vi "rszvl_core_global.vi"() -> ()   [LabVIEW 2014] (continued)
  in  "Range Tables":T3(array[cluster])=[{"Name"="rszvl_rngUnits", "Type"=2, "Min?"=FALSE, "Max?"=FALSE, "Entries"=[{"Name"="RSZVL_VAL_UNIT_DBM", "Discrete or Min"=0.0, "Max"=0.0, "Coerced"=0.0, "Command"="DBM"}, {"Name"="RSZVL_VAL_UNIT_DBPW", "Discrete or Min"=1.0, "Max"=0.0, "Coerced"=0.0, "Command"="DBPW"}, {"Name"="RSZVL_VAL_UNIT_WATT", "Discrete or Min"=2.0, "Max"=0.0, "Coerced"=0.0, "Command"="WATT"}, {"Name"="RSZVL_VAL_UNIT_DBUV", "Discrete or Min"=3.0, "Max"=0.0, "Coerced"=0.0, "Command"="DBUV"}, {"Name"="RSZVL_VAL_UNIT_DBMV", "Discrete or Min"=4.0, "Max"=0.0, "Coerced"=0.0, "Command"="DBMV"}, {"Name"="RSZVL_VAL_UNIT_VOLT", "Discrete or Min"=5.0, "Max"=0.0, "Coerced"=0.0, "Command"="VOLT"}, {"Name"="RSZVL_VAL_UNIT_DBUA", "Discrete or Min"=6.0, "Max"=0.0, "Coerced"=0.0, "Command"="DBUA"}, {"Name"="RSZVL_VAL_UNIT_AMP", "Discrete or Min"=7.0, "Max"=0.0, "Coerced"=0.0, "Command"="AMP"}, {"Name"="RSZVL_VAL_UNIT_DB", "Discrete or Min"=8.0, "Max"=0.0, "Coerced"=0.0, "Command"="DB"}, {"Name"="RSZVL_VAL_UNIT_DEG", "Discrete or Min"=9.0, "Max"=0.0, "Coerced"=0.0, "Command"="DEG"}, {"Name"="RSZVL_VAL_UNIT_RAD", "Discrete or Min"=10.0, "Max"=0.0, "Coerced"=0.0, "Command"="RAD"}, {"Name"="RSZVL_VAL_UNIT_S", "Discrete or Min"=11.0, "Max"=0.0, "Coerced"=0.0, "Command"="S"}, {"Name"="RSZVL_VAL_UNIT_HZ", "Discrete or Min"=12.0, "Max"=0.0, "Coerced"=0.0, "Command"="HZ"}, {"Name"="RSZVL_VAL_UNIT_PCT", "Discrete or Min"=13.0, "Max"=0.0, "Coerced"=0.0, "Command"="PCT"}, {"Name"="RSZVL_VAL_UNIT_UNITLESS", "Discrete or Min"=14.0, "Max"=0.0, "Coerced"=0.0, "Command"="UNIT"}, {"Name"="RSZVL_VAL_UNIT_DBPT", "Discrete or Min"=15.0, "Max"=0.0, "Coerced"=0.0, "Command"="DBPT"}]}, {"Name"="rszvl_rngTraceMode", "Type"=2, "Min?"=FALSE, "Max?"=FALSE, "Entries"=[{"Name"="RSZVL_TRAC_MOD_WRITE", "Discrete or Min"=0.0, "Max"=0.0, "Coerced"=0.0, "Command"="WRIT"}, {"Name"="RSZVL_TRAC_MOD_VIEW", "Discrete or Min"=1.0, "Max"=0.0, "Coerced"=0.0, "Command"="VIEW"}, {"Name"="RSZVL_TRAC_MOD_AVER", "Discrete or Min"=2.0, "Max"=0.0, "Coerced"=0.0, "Command"="AVER"}, {"Name"="RSZVL_TRAC_MOD_MAXH", "Discrete or Min"=3.0, "Max"=0.0, "Coerced"=0.0, "Command"="MAXH"}, {"Name"="RSZVL_TRAC_MOD_MINH", "Discrete or Min"=4.0, "Max"=0.0, "Coerced"=0.0, "Command"="MINH"}, {"Name"="RSZVL_TRAC_MOD_BLANK", "Discrete or Min"=5.0, "Max"=0.0, "Coerced"=0.0, "Command"="BLAN"}]}, {"Name"="rszvl_rngAmplitudeUnitsRangeTable", "Type"=2, "Min?"=FALSE, "Max?"=FALSE, "Entries"=[{"Name"="RSZVL_VAL_AMPLITUDE_UNITS_DBM", "Discrete or Min"=0.0, "Max"=0.0, "Coerced"=0.0, "Command"="DBM"}, {"Name"="RSZVL_VAL_AMPLITUDE_UNITS_DBMV", "Discrete or Min"=1.0, "Max"=0.0, "Coerced"=0.0, "Command"="DBMV"}, {"Name"="RSZVL_VAL_AMPLITUDE_UNITS_DBUV", "Discrete or Min"=2.0, "Max"=0.0, "Coerced"=0.0, "Command"="DBUV"}, {"Name"="RSZVL_VAL_AMPLITUDE_UNITS_VOLT", "Discrete or Min"=3.0, "Max"=0.0, "Coerced"=0.0, "Command"="V"}, {"Name"="RSZVL_VAL_AMPLITUDE_UNITS_WATT", "Discrete or Min"=4.0, "Max"=0.0, "Coerced"=0.0, "Command"="W"}, {"Name"="RSZVL_VAL_AMPLITUDE_UNITS_DBPW", "Discrete or Min"=5.0, "Max"=0.0, "Coerced"=0.0, "Command"="DBPW"}, {"Name"="RSZVL_VAL_AMPLITUDE_UNITS_DBUA", "Discrete or Min"=6.0, "Max"=0.0, "Coerced"=0.0, "Command"="DBUA"}, {"Name"="RSZVL_VAL_AMPLITUDE_UNITS_AMP", "Discrete or Min"=7.0, "Max"=0.0, "Coerced"=0.0, "Command"="A"}]}, {"Name"="rszvl_rngAbsRel", "Type"=2, "Min?"=FALSE, "Max?"=FALSE, "Entries"=[{"Name"="RSZVL_VAL_ABS", "Discrete or Min"=0.0, "Max"=0.0, "Coerced"=0.0, "Command"="ABS"}, {"Name"="RSZVL_VAL_REL", "Discrete or Min"=1.0, "Max"=0.0, "Coerced"=0.0, "Command"="REL"}]}, {"Name"="rszvl_rngESPMode", "Type"=2, "Min?"=FALSE, "Max?"=FALSE, "Entries"=[{"Name"="RSZVL_VAL_ESP_MODE_AUTO", "Discrete or Min"=0.0, "Max"=0.0, "Coerced"=0.0, "Command"="AUTO"}, {"Name"="RSZVL_VAL_ESP_MODE_MAN", "Discrete or Min"=1.0, "Max"=0.0, "Coerced"=0.0, "Command"="MAN"}, {"Name"="RSZVL_VAL_ESP_MODE_USER", "Discrete or Min"=2.0, "Max"=0.0, "Coerced"=0.0, "Command"="USER"}]}, {"Name"="rszvl_rngDetectorTypeRangeTable", "Type"=2, "Min?"=FALSE, "Max?"=FALSE, "Entries"=[{"Name"="RSZVL_VAL_DETECTOR_TYPE_AUTO_PEAK", "Discrete or Min"=0.0, "Max"=0.0, "Coerced"=0.0, "Command"="APE"}, {"Name"="RSZVL_VAL_DETECTOR_TYPE_AVERAGE", "Discrete or Min"=1.0, "Max"=0.0, "Coerced"=0.0, "Command"="AVER"}, {"Name"="RSZVL_VAL_DETECTOR_TYPE_MAX_PEAK", "Discrete or Min"=2.0, "Max"=0.0, "Coerced"=0.0, "Command"="POS"}, {"Name"="RSZVL_VAL_DETECTOR_TYPE_MIN_PEAK", "Discrete or Min"=3.0, "Max"=0.0, "Coerced"=0.0, "Command"="NEG"}, {"Name"="RSZVL_VAL_DETECTOR_TYPE_SAMPLE", "Discrete or Min"=4.0, "Max"=0.0, "Coerced"=0.0, "Command"="SAMP"}, {"Name"="RSZVL_VAL_DETECTOR_TYPE_RMS", "Discrete or Min"=5.0, "Max"=0.0, "Coerced"=0.0, "Command"="RMS"}, {"Name"="RSZVL_VAL_DETECTOR_TYPE_QPK", "Discrete or Min"=6.0, "Max"=0.0, "Coerced"=0.0, "Command"="QPE"}]}, {"Name"="rszvl_rngDISPConfPreDefColour", "Type"=2, "Min?"=FALSE, "Max?"=FALSE, "Entries"=[{"Name"="RSZVL_VAL_DISP_COL_BLAC", "Discrete or Min"=0.0, "Max"=0.0, "Coerced"=0.0, "Command"="BLAC"}, {"Name"="RSZVL_VAL_DISP_COL_BLUE", "Discrete or Min"=1.0, "Max"=0.0, "Coerced"=0.0, "Command"="BLUE"}, {"Name"="RSZVL_VAL_DISP_COL_BROW", "Discrete or Min"=2.0, "Max"=0.0, "Coerced"=0.0, "Command"="BROW"}, {"Name"="RSZVL_VAL_DISP_COL_GRE", "Discrete or Min"=3.0, "Max"=0.0, "Coerced"=0.0, "Command"="GRE"}, {"Name"="RSZVL_VAL_DISP_COL_CYAN", "Discrete or Min"=4.0, "Max"=0.0, "Coerced"=0.0, "Command"="CYAN"}, {"Name"="RSZVL_VAL_DISP_COL_RED", "Discrete or Min"=5.0, "Max"=0.0, "Coerced"=0.0, "Command"="RED"}, {"Name"="RSZVL_VAL_DISP_COL_MAG", "Discrete or Min"=6.0, "Max"=0.0, "Coerced"=0.0, "Command"="MAG"}, {"Name"="RSZVL_VAL_DISP_COL_YELL", "Discrete or Min"=7.0, "Max"=0.0, "Coerced"=0.0, "Command"="YELL"}, {"Name"="RSZVL_VAL_DISP_COL_WHIT", "Discrete or Min"=8.0, "Max"=0.0, "Coerced"=0.0, "Command"="WHIT"}, {"Name"="RSZVL_VAL_DISP_COL_DGRA", "Discrete or Min"=9.0, "Max"=0.0, "Coerced"=0.0, "Command"="DGR"}, {"Name"="RSZVL_VAL_DISP_COL_LGRA", "Discrete or Min"=10.0, "Max"=0.0, "Coerced"=0.0, "Command"="LGR"}, {"Name"="RSZVL_VAL_DISP_COL_LBLU", "Discrete or Min"=11.0, "Max"=0.0, "Coerced"=0.0, "Command"="LBL"}, {"Name"="RSZVL_VAL_DISP_COL_LGRE", "Discrete or Min"=12.0, "Max"=0.0, "Coerced"=0.0, "Command"="LGR"}, {"Name"="RSZVL_VAL_DISP_COL_LCY", "Discrete or Min"=13.0, "Max"=0.0, "Coerced"=0.0, "Command"="LCY"}, {"Name"="RSZVL_VAL_DISP_COL_LRED", "Discrete or Min"=14.0, "Max"=0.0, "Coerced"=0.0, "Command"="LRED"}, {"Name"="RSZVL_VAL_DISP_COL_LMAG", "Discrete or Min"=15.0, "Max"=0.0, "Coerced"=0.0, "Command"="LMAG"}]}, {"Name"="rszvl_rngHcopyDeviceLang", "Type"=2, "Min?"=FALSE, "Max?"=FALSE, "Entries"=[{"Name"="RSZVL_VAL_HCOPY_DEVICE_LANG_GDI", "Discrete or Min"=0.0, "Max"=0.0, "Coerced"=0.0, "Command"="GDI"}, {"Name"="RSZVL_VAL_HCOPY_DEVICE_LANG_WMF", "Discrete or Min"=1.0, "Max"=0.0, "Coerced"=0.0, "Command"="WMF"}, {"Name"="RSZVL_VAL_HCOPY_DEVICE_LANG_EWMF", "Discrete or Min"=2.0, "Max"=0.0, "Coerced"=0.0, "Command"="EWMF"}, {"Name"="RSZVL_VAL_HCOPY_DEVICE_LANG_BMP", "Discrete or Min"=3.0, "Max"=0.0, "Coerced"=0.0, "Command"="BMP"}, {"Name"="RSZVL_VAL_HCOPY_DEVICE_LANG_JPG", "Discrete or Min"=4.0, "Max"=0.0, "Coerced"=0.0, "Command"="JPG"}, {"Name"="RSZVL_VAL_HCOPY_DEVICE_LANG_PNG", "Discrete or Min"=5.0, "Max"=0.0, "Coerced"=0.0, "Command"="PNG"}]}, {"Name"="rszvl_rngHcopyDeviceOrient", "Type"=2, "Min?"=FALSE, "Max?"=FALSE, "Entries"=[{"Name"="RSZVL_VAL_HCOPY_DEVICE_ORIENT_LAND", "Discrete or Min"=0.0, "Max"=0.0, "Coerced"=0.0, "Command"="LAND"}, {"Name"="RSZVL_VAL_HCOPY_DEVICE_ORIENT_PORT", "Discrete or Min"=1.0, "Max"=0.0, "Coerced"=0.0, "Command"="PORT"}]}, {"Name"="rszvl_rngDomain", "Type"=2, "Min?"=FALSE, "Max?"=FALSE, "Entries"=[{"Name"="RSZVL_VAL_FREQ", "Discrete or Min"=0.0, "Max"=0.0, "Coerced"=0.0, "Command"="FREQ"}, {"Name"="RSZVL_VAL_TIME", "Discrete or Min"=1.0, "Max"=0.0, "Coerced"=0.0, "Command"="TIME"}]}, {"Name"="rszvl_rngLinLog", "Type"=2, "Min?"=FALSE, "Max?"=FALSE, "Entries"=[{"Name"="RSZVL_VAL_VBW_FILT_LIN", "Discrete or Min"=0.0, "Max"=0.0, "Coerced"=0.0, "Command"="LIN"}, {"Name"="RSZVL_VAL_VBW_FILT_LOG", "Discrete or Min"=1.0, "Max"=0.0, "Coerced"=0.0, "Command"="LOG"}]}, {"Name"="rszvl_rngServiceInput", "Type"=2, "Min?"=FALSE, "Max?"=FALSE, "Entries"=[{"Name"="RSZVL_VAL_INPUT_RF", "Discrete or Min"=0.0, "Max"=0.0, "Coerced"=0.0, "Command"="RF"}, {"Name"="RSZVL_VAL_INPUT_CAL", "Discrete or Min"=1.0, "Max"=0.0, "Coerced"=0.0, "Command"="CAL"}, {"Name"="RSZVL_VAL_INPUT_TG", "Discrete or Min"=2.0, "Max"=0.0, "Coerced"=0.0, "Command"="TG"}]}, {"Name"="rszvl_rngAvgType", "Type"=2, "Min?"=FALSE, "Max?"=FALSE, "Entries"=[{"Name"="RSZVL_VAL_AVG_LIN", "Discrete or Min"=0.0, "Max"=0.0, "Coerced"=0.0, "Command"="LIN"}, {"Name"="RSZVL_VAL_AVG_VID", "Discrete or Min"=1.0, "Max"=0.0, "Coerced"=0.0, "Command"="VID"}]}, {"Name"="rszvl_rngDISPSizeWindow", "Type"=2, "Min?"=FALSE, "Max?"=FALSE, "Entries"=[{"Name"="RSZVL_VAL_DISP_SIZE_LARGE", "Discrete or Min"=0.0, "Max"=0.0, "Coerced"=0.0, "Command"="LARG"}, {"Name"="RSZVL_VAL_DISP_SIZE_SMALL", "Discrete or Min"=1.0, "Max"=0.0, "Coerced"=0.0, "Command"="SMAL"}]}, {"Name"="rszvl_rngMarkerPeakListSort", "Type"=2, "Min?"=FALSE, "Max?"=FALSE, "Entries"=[{"Name"="RSZVL_VAL_MARKER_SORT_X", "Discrete or Min"=0.0, "Max"=0.0, "Coerced"=0.0, "Command"="X"}, {"Name"="RSZVL_VAL_MARKER_SORT_Y", "Discrete or Min"=1.0, "Max"=0.0, "Coerced"=0.0, "Command"="Y"}]}, {"Name"="rszvl_rngMarkerDemodType", "Type"=2, "Min?"=FALSE, "Max?"=FALSE, "Entries"=[{"Name"="RSZVL_VAL_MARKER_DEMOD_AM", "Discrete or Min"=0.0, "Max"=0.0, "Coerced"=0.0, "Command"="AM"}, {"Name"="RSZVL_VAL_MARKER_DEMOD_FM", "Discrete or Min"=1.0, "Max"=0.0, "Coerced"=0.0, "Command"="FM"}]}, {"Name"="rszvl_rngMeasPowerSelect", "Type"=2, "Min?"=FALSE, "Max?"=FALSE, "Entries"=[{"Name"="RSZVL_VAL_MEAS_POW_ACP", "Discrete or Min"=0.0, "Max"=0.0, "Coerced"=0.0, "Command"="ACP"}, {"Name"="RSZVL_VAL_MEAS_POW_CPOW", "Discrete or Min"=1.0, "Max"=0.0, "Coerced"=0.0, "Command"="CPOW"}, {"Name"="RSZVL_VAL_MEAS_POW_MCAC", "Discrete or Min"=2.0, "Max"=0.0, "Coerced"=0.0, "Command"="MCAC"}, {"Name"="RSZVL_VAL_MEAS_POW_OBAN", "Discrete or Min"=3.0, "Max"=0.0, "Coerced"=0.0, "Command"="OBAN"}, {"Name"="RSZVL_VAL_MEAS_POW_CN", "Discrete or Min"=4.0, "Max"=0.0, "Coerced"=0.0, "Command"="CN"}, {"Name"="RSZVL_VAL_MEAS_POW_CN0", "Discrete or Min"=5.0, "Max"=0.0, "Coerced"=0.0, "Command"="CN0"}]}, {"Name"="rszvl_rngMeasPowerStandard", "Type"=2, "Min?"=FALSE, "Max?"=FALSE, "Entries"=[{"Name"="RSZVL_VAL_MEAS_POW_STD_NONE", "Discrete or Min"=0.0, "Max"=0.0, "Coerced"=0.0, "Command"="NONE"}, {"Name"="RSZVL_VAL_MEAS_POW_STD_NADC", "Discrete or Min"=1.0, "Max"=0.0, "Coerced"=0.0, "Command"="NADC"}, {"Name"="RSZVL_VAL_MEAS_POW_STD_TETRA", "Discrete or Min"=2.0, "Max"=0.0, "Coerced"=0.0, "Command"="TETRA"}, {"Name"="RSZVL_VAL_MEAS_POW_STD_PDC", "Discrete or Min"=3.0, "Max"=0.0, "Coerced"=0.0, "Command"="PDC"}, {"Name"="RSZVL_VAL_MEAS_POW_STD_PHS", "Discrete or Min"=4.0, "Max"=0.0, "Coerced"=0.0, "Command"="PHS"}, {"Name"="RSZVL_VAL_MEAS_POW_STD_CDPD", "Discrete or Min"=5.0, "Max"=0.0, "Coerced"=0.0, "Command"="CDPD"}, {"Name"="RSZVL_VAL_MEAS_POW_STD_FIS95A", "Discrete or Min"=6.0, "Max"=0.0, "Coerced"=0.0, "Command"="F8CD"}, {"Name"="RSZVL_VAL_MEAS_POW_STD_RIS95A", "Discrete or Min"=7.0, "Max"=0.0, "Coerced"=0.0, "Command"="R8CD"}, {"Name"="RSZVL_VAL_MEAS_POW_STD_FIS95C0", "Discrete or Min"=8.0, "Max"=0.0, "Coerced"=0.0, "Command"="FIS95C0"}, {"Name"="RSZVL_VAL_MEAS_POW_STD_RIS95C0", "Discrete or Min"=9.0, "Max"=0.0, "Coerced"=0.0, "Command"="RIS95C0"}, {"Name"="RSZVL_VAL_MEAS_POW_STD_FJ008", "Discrete or Min"=10.0, "Max"=0.0, "Coerced"=0.0, "Command"="F19C"}, {"Name"="RSZVL_VAL_MEAS_POW_STD_RJ008", "Discrete or Min"=11.0, "Max"=0.0, "Coerced"=0.0, "Command"="R19C"}, {"Name"="RSZVL_VAL_MEAS_POW_STD_FIS95C1", "Discrete or Min"=12.0, "Max"=0.0, "Coerced"=0.0, "Command"="FIS95C1"}, {"Name"="RSZVL_VAL_MEAS_POW_STD_RIS95C1", "Discrete or Min"=13.0, "Max"=0.0, "Coerced"=0.0, "Command"="RIS95C1"}, {"Name"="RSZVL_VAL_MEAS_POW_STD_FWCD", "Discrete or Min"=14.0, "Max"=0.0, "Coerced"=0.0, "Command"="FWCD"}, {"Name"="RSZVL_VAL_MEAS_POW_STD_RWCD", "Discrete or Min"=15.0, "Max"=0.0, "Coerced"=0.0, "Command"="RWCD"}, {"Name"="RSZVL_VAL_MEAS_POW_STD_FW3G", "Discrete or Min"=16.0, "Max"=0.0, "Coerced"=0.0, "Command"="FW3G"}, {"Name"="RSZVL_VAL_MEAS_POW_STD_RW3G", "Discrete or Min"=17.0, "Max"=0.0, "Coerced"=0.0, "Command"="RW3G"}, {"Name"="RSZVL_VAL_MEAS_POW_STD_D2CD", "Discrete or Min"=18.0, "Max"=0.0, "Coerced"=0.0, "Command"="D2CD"}, {"Name"="RSZVL_VAL_MEAS_POW_STD_S2CD", "Discrete or Min"=19.0, "Max"=0.0, "Coerced"=0.0, "Command"="S2CD"}, {"Name"="RSZVL_VAL_MEAS_POW_STD_M2CD", "Discrete or Min"=20.0, "Max"=0.0, "Coerced"=0.0, "Command"="M2CD"}, {"Name"="RSZVL_VAL_MEAS_POW_STD_TCDM", "Discrete or Min"=21.0, "Max"=0.0, "Coerced"=0.0, "Command"="TCDM"}, {"Name"="RSZVL_VAL_MEAS_POW_STD_AWL", "Discrete or Min"=22.0, "Max"=0.0, "Coerced"=0.0, "Command"="AWLAN"}, {"Name"="RSZVL_VAL_MEAS_POW_STD_BWL", "Discrete or Min"=23.0, "Max"=0.0, "Coerced"=0.0, "Command"="BWLAN"}, {"Name"="RSZVL_VAL_MEAS_POW_STD_WIM", "Discrete or Min"=24.0, "Max"=0.0, "Coerced"=0.0, "Command"="WIMax"}, {"Name"="RSZVL_VAL_MEAS_POW_STD_WIBRO", "Discrete or Min"=25.0, "Max"=0.0, "Coerced"=0.0, "Command"="WIBRo"}]}, {"Name"="rszvl_rngMeasPowerMode", "Type"=2, "Min?"=FALSE, "Max?"=FALSE, "Entries"=[{"Name"="RSZVL_VAL_MEAS_POW_MODE_WRITE", "Discrete or Min"=0.0, "Max"=0.0, "Coerced"=0.0, "Command"="WRIT"}, {"Name"="RSZVL_VAL_MEAS_POW_MODE_MAXH", "Discrete or Min"=1.0, "Max"=0.0, "Coerced"=0.0, "Command"="MAXH"}]}, {"Name"="rszvl_rngBandFiltType", "Type"=2, "Min?"=FALSE, "Max?"=FALSE, "Entries"=[{"Name"="RSZVL_VAL_FILT_TYPE_NORM", "Discrete or Min"=0.0, "Max"=0.0, "Coerced"=0.0, "Command"="NORM"}, {"Name"="RSZVL_VAL_FILT_TYPE_FFT", "Discrete or Min"=1.0, "Max"=0.0, "Coerced"=0.0, "Command"="FFT"}, {"Name"="RSZVL_VAL_FILT_TYPE_CFIL", "Discrete or Min"=2.0, "Max"=0.0, "Coerced"=0.0, "Command"="CFIL"}, {"Name"="RSZVL_VAL_FILT_TYPE_RRC", "Discrete or Min"=3.0, "Max"=0.0, "Coerced"=0.0, "Command"="RRC"}, {"Name"="RSZVL_VAL_FILT_TYPE_PULSE", "Discrete or Min"=4.0, "Max"=0.0, "Coerced"=0.0, "Command"="PULS"}]}, {"Name"="rszvl_rngTFacUnit", "Type"=2, "Min?"=FALSE, "Max?"=FALSE, "Entries"=[{"Name"="RSZVL_VAL_TFAC_UNIT_DB", "Discrete or Min"=0.0, "Max"=0.0, "Coerced"=0.0, "Command"="DB"}, {"Name"="RSZVL_VAL_TFAC_UNIT_DBM", "Discrete or Min"=1.0, "Max"=0.0, "Coerced"=0.0, "Command"="DBM"}, {"Name"="RSZVL_VAL_TFAC_UNIT_DBMV", "Discrete or Min"=2.0, "Max"=0.0, "Coerced"=0.0, "Command"="DBMV"}, {"Name"="RSZVL_VAL_TFAC_UNIT_DBUV", "Discrete or Min"=3.0, "Max"=0.0, "Coerced"=0.0, "Command"="DBUV"}, {"Name"="RSZVL_VAL_TFAC_UNIT_DBUVM", "Discrete or Min"=4.0, "Max"=0.0, "Coerced"=0.0, "Command"="DBUV/M"}, {"Name"="RSZVL_VAL_TFAC_UNIT_DBUA", "Discrete or Min"=5.0, "Max"=0.0, "Coerced"=0.0, "Command"="DBUA"}, {"Name"="RSZVL_VAL_TFAC_UNIT_DBUAM", "Discrete or Min"=6.0, "Max"=0.0, "Coerced"=0.0, "Command"="DBUA/M"}, {"Name"="RSZVL_VAL_TFAC_UNIT_DBPW", "Discrete or Min"=7.0, "Max"=0.0, "Coerced"=0.0, "Command"="DBPW"}, {"Name"="RSZVL_VAL_TFAC_UNIT_DBPT", "Discrete or Min"=8.0, "Max"=0.0, "Coerced"=0.0, "Command"="DBPT"}]}, {"Name"="rszvl_rngFreqCentLink", "Type"=2, "Min?"=FALSE, "Max?"=FALSE, "Entries"=[{"Name"="RSZVL_VAL_CENT_FREQ_LINK_OFF", "Discrete or Min"=0.0, "Max"=0.0, "Coerced"=0.0, "Command"="OFF"}, {"Name"="RSZVL_VAL_CENT_FREQ_LINK_SPAN", "Discrete or Min"=1.0, "Max"=0.0, "Coerced"=0.0, "Command"="SPAN"}, {"Name"="RSZVL_VAL_CENT_FREQ_LINK_RBW", "Discrete or Min"=2.0, "Max"=0.0, "Coerced"=0.0, "Command"="RBW"}]}, {"Name"="rszvl_rngFreqMode", "Type"=2, "Min?"=FALSE, "Max?"=FALSE, "Entries"=[{"Name"="RSZVL_VAL_FREQ_MODE_CW", "Discrete or Min"=0.0, "Max"=0.0, "Coerced"=0.0, "Command"="CW"}, {"Name"="RSZVL_VAL_FREQ_MODE_FIX", "Discrete or Min"=1.0, "Max"=0.0, "Coerced"=0.0, "Command"="FIX"}, {"Name"="RSZVL_VAL_FREQ_MODE_SWE", "Discrete or Min"=2.0, "Max"=0.0, "Coerced"=0.0, "Command"="SWE"}]}, {"Name"="rszvl_rngOffOnAuto", "Type"=2, "Min?"=FALSE, "Max?"=FALSE, "Entries"=[{"Name"="RSZVL_VAL_STATE_OFF", "Discrete or Min"=0.0, "Max"=0.0, "Coerced"=0.0, "Command"="OFF"}, {"Name"="RSZVL_VAL_STATE_ON", "Discrete or Min"=1.0, "Max"=0.0, "Coerced"=0.0, "Command"="ON"}, {"Name"="RSZVL_VAL_STATE_AUTO", "Discrete or Min"=2.0, "Max"=0.0, "Coerced"=0.0, "Command"="AUTO"}]}, {"Name"="rszvl_rngExtMixerHarmonicType", "Type"=2, "Min?"=FALSE, "Max?"=FALSE, "Entries"=[{"Name"="RSZVL_VAL_EXT_MIX_HARM_ODD", "Discrete or Min"=0.0, "Max"=0.0, "Coerced"=0.0, "Command"="ODD"}, {"Name"="RSZVL_VAL_EXT_MIX_HARM_EVEN", "Discrete or Min"=1.0, "Max"=0.0, "Coerced"=0.0, "Command"="EVEN"}, {"Name"="RSZVL_VAL_EXT_MIX_HARM_EODD", "Discrete or Min"=2.0, "Max"=0.0, "Coerced"=0.0, "Command"="EODD"}]}, {"Name"="rszvl_rngExtMixerHarmBand", "Type"=2, "Min?"=FALSE, "Max?"=FALSE, "Entries"=[{"Name"="RSZVL_VAL_EXT_MIX_BAND_A", "Discrete or Min"=0.0, "Max"=0.0, "Coerced"=0.0, "Command"="A"}, {"Name"="RSZVL_VAL_EXT_MIX_BAND_Q", "Discrete or Min"=1.0, "Max"=0.0, "Coerced"=0.0, "Command"="Q"}, {"Name"="RSZVL_VAL_EXT_MIX_BAND_U", "Discrete or Min"=2.0, "Max"=0.0, "Coerced"=0.0, "Command"="U"}, {"Name"="RSZVL_VAL_EXT_MIX_BAND_V", "Discrete or Min"=3.0, "Max"=0.0, "Coerced"=0.0, "Command"="V"}, {"Name"="RSZVL_VAL_EXT_MIX_BAND_E", "Discrete or Min"=4.0, "Max"=0.0, "Coerced"=0.0, "Command"="E"}, {"Name"="RSZVL_VAL_EXT_MIX_BAND_W", "Discrete or Min"=5.0, "Max"=0.0, "Coerced"=0.0, "Command"="W"}, {"Name"="RSZVL_VAL_EXT_MIX_BAND_F", "Discrete or Min"=6.0, "Max"=0.0, "Coerced"=0.0, "Command"="F"}, {"Name"="RSZVL_VAL_EXT_MIX_BAND_D", "Discrete or Min"=7.0, "Max"=0.0, "Coerced"=0.0, "Command"="D"}, {"Name"="RSZVL_VAL_EXT_MIX_BAND_G", "Discrete or Min"=8.0, "Max"=0.0, "Coerced"=0.0, "Command"="G"}, {"Name"="RSZVL_VAL_EXT_MIX_BAND_Y", "Discrete or Min"=9.0, "Max"=0.0, "Coerced"=0.0, "Command"="Y"}, {"Name"="RSZVL_VAL_EXT_MIX_BAND_J", "Discrete or Min"=10.0, "Max"=0.0, "Coerced"=0.0, "Command"="J"}, {"Name"="RSZVL_VAL_EXT_MIX_BAND_USER", "Discrete or Min"=11.0, "Max"=0.0, "Coerced"=0.0, "Command"="USER"}]}, {"Name"="rszvl_rngAdjChAutoSel", "Type"=2, "Min?"=FALSE, "Max?"=FALSE, "Entries"=[{"Name"="RSZVL_VAL_ADJ_RCHAN_AUTO_MIN", "Discrete or Min"=0.0, "Max"=0.0, "Coerced"=0.0, "Command"="MIN"}, {"Name"="RSZVL_VAL_ADJ_RCHAN_AUTO_MAX", "Discrete or Min"=1.0, "Max"=0.0, "Coerced"=0.0, "Command"="MAX"}, {"Name"="RSZVL_VAL_ADJ_RCHAN_AUTO_LHIG", "Discrete or Min"=2.0, "Max"=0.0, "Coerced"=0.0, "Command"="LHIG"}]}, {"Name"="rszvl_rngAdjPreset", "Type"=2, "Min?"=FALSE, "Max?"=FALSE, "Entries"=[{"Name"="RSZVL_VAL_ADJ_PRE_ACP", "Discrete or Min"=0.0, "Max"=0.0, "Coerced"=0.0, "Command"="ACP"}, {"Name"="RSZVL_VAL_ADJ_PRE_CPOW", "Discrete or Min"=1.0, "Max"=0.0, "Coerced"=0.0, "Command"="CPOW"}, {"Name"="RSZVL_VAL_ADJ_PRE_MCAC", "Discrete or Min"=2.0, "Max"=0.0, "Coerced"=0.0, "Command"="MCAC"}, {"Name"="RSZVL_VAL_ADJ_PRE_OBAN", "Discrete or Min"=3.0, "Max"=0.0, "Coerced"=0.0, "Command"="OBAN"}, {"Name"="RSZVL_VAL_ADJ_PRE_CN", "Discrete or Min"=4.0, "Max"=0.0, "Coerced"=0.0, "Command"="CN"}, {"Name"="RSZVL_VAL_ADJ_PRE_CN0", "Discrete or Min"=5.0, "Max"=0.0, "Coerced"=0.0, "Command"="CN0"}]}, {"Name"="rszvl_rngSourceIntExt", "Type"=2, "Min?"=FALSE, "Max?"=FALSE, "Entries"=[{"Name"="RSZVL_VAL_SOUR_INT", "Discrete or Min"=0.0, "Max"=0.0, "Coerced"=0.0, "Command"="INT"}, {"Name"="RSZVL_VAL_SOUR_EXT", "Discrete or Min"=1.0, "Max"=0.0, "Coerced"=0.0, "Command"="EXT"}]}, {"Name"="rszvl_rngExtGateTrigType", "Type"=2, "Min?"=FALSE, "Max?"=FALSE, "Entries"=[{"Name"="RSZVL_VAL_EGAT_TRIG_LEV", "Discrete or Min"=0.0, "Max"=0.0, "Coerced"=0.0, "Command"="LEV"}, {"Name"="RSZVL_VAL_EGAT_TRIG_EDGE", "Discrete or Min"=1.0, "Max"=0.0, "Coerced"=0.0, "Command"="EDGE"}]}, {"Name"="rszvl_rngHcopyDevice", "Type"=2, "Min?"=FALSE, "Max?"=FALSE, "Entries"=[{"Name"="RSZVL_VAL_HCOPY_DEVICE_MEM", "Discrete or Min"=0.0, "Max"=0.0, "Coerced"=0.0, "Command"="'MMEM'"}, {"Name"="RSZVL_VAL_HCOPY_DEVICE_PRN", "Discrete or Min"=1.0, "Max"=0.0, "Coerced"=0.0, "Command"="'SYST:COMM:PRIN'"}, {"Name"="RSZVL_VAL_HCOPY_DEVICE_CLP", "Discrete or Min"=2.0, "Max"=0.0, "Coerced"=0.0, "Command"="'SYST:COMM:CLIP'"}]}, {"Name"="rszvl_rngPolarity", "Type"=2, "Min?"=FALSE, "Max?"=FALSE, "Entries"=[{"Name"="RSZVL_VAL_NEG", "Discrete or Min"=0.0, "Max"=0.0, "Coerced"=0.0, "Command"="NEG"}, {"Name"="RSZVL_VAL_POS", "Discrete or Min"=1.0, "Max"=0.0, "Coerced"=0.0, "Command"="POS"}]}, {"Name"="rszvl_rngExtGateSource", "Type"=2, "Min?"=FALSE, "Max?"=FALSE, "Entries"=[{"Name"="RSZVL_VAL_EGAT_SOUR_EXT", "Discrete or Min"=0.0, "Max"=0.0, "Coerced"=0.0, "Command"="EXT"}, {"Name"="RSZVL_VAL_EGAT_SOUR_IFP", "Discrete or Min"=1.0, "Max"=0.0, "Coerced"=0.0, "Command"="IFP"}]}, {"Name"="rszvl_rngSweepContMode", "Type"=2, "Min?"=FALSE, "Max?"=FALSE, "Entries"=[{"Name"="RSZVL_VAL_SWE_MODE_AUTO", "Discrete or Min"=0.0, "Max"=0.0, "Coerced"=0.0, "Command"="AUTO"}, {"Name"="RSZVL_VAL_SWE_MODE_LIST", "Discrete or Min"=1.0, "Max"=0.0, "Coerced"=0.0, "Command"="LIST"}, {"Name"="RSZVL_VAL_SWE_MODE_ESYNC", "Discrete or Min"=2.0, "Max"=0.0, "Coerced"=0.0, "Command"="ESYNC"}]}, {"Name"="rszvl_rngTriggerSource", "Type"=2, "Min?"=FALSE, "Max?"=FALSE, "Entries"=[{"Name"="RSZVL_VAL_TRG_IMM", "Discrete or Min"=0.0, "Max"=0.0, "Coerced"=0.0, "Command"="IMM"}, {"Name"="RSZVL_VAL_TRG_EXT", "Discrete or Min"=1.0, "Max"=0.0, "Coerced"=0.0, "Command"="EXT"}, {"Name"="RSZVL_VAL_TRG_IFP", "Discrete or Min"=2.0, "Max"=0.0, "Coerced"=0.0, "Command"="IFP"}, {"Name"="RSZVL_VAL_TRG_VID", "Discrete or Min"=3.0, "Max"=0.0, "Coerced"=0.0, "Command"="VID"}, {"Name"="RSZVL_VAL_TRG_TIME", "Discrete or Min"=4.0, "Max"=0.0, "Coerced"=0.0, "Command"="TIME"}]}, {"Name"="rszvl_rngFileDecSeparator", "Type"=2, "Min?"=FALSE, "Max?"=FALSE, "Entries"=[{"Name"="RSZVL_VAL_DEC_SEP_POIN", "Discrete or Min"=0.0, "Max"=0.0, "Coerced"=0.0, "Command"="POIN"}, {"Name"="RSZVL_VAL_DEC_SEP_COMMA", "Discrete or Min"=1.0, "Max"=0.0, "Coerced"=0.0, "Command"="COMM"}]}, {"Name"="rszvl_rngCalibration", "Type"=0, "Min?"=TRUE, "Max?"=TRUE, "Entries"=[{"Name"="", "Discrete or Min"=0.0, "Max"=1.0, "Coerced"=0.0, "Command"=""}]}, {"Name"="rszvl_rngMarkerStepSize", "Type"=2, "Min?"=FALSE, "Max?"=FALSE, "Entries"=[{"Name"="RSZVL_VAL_MARK_STEP_SIZE_STAN", "Discrete or Min"=0.0, "Max"=0.0, "Coerced"=0.0, "Command"="STAN"}, {"Name"="RSZVL_VAL_MARK_STEP_SIZE_POIN", "Discrete or Min"=1.0, "Max"=0.0, "Coerced"=0.0, "Command"="POIN"}]}, {"Name"="rszvl_rngMpowFiltType", "Type"=2, "Min?"=FALSE, "Max?"=FALSE, "Entries"=[{"Name"="RSZVL_VAL_MPOW_FTYPE_NORM", "Discrete or Min"=0.0, "Max"=0.0, "Coerced"=0.0, "Command"="NORM"}, {"Name"="RSZVL_VAL_MPOW_FTYPE_CFIL", "Discrete or Min"=1.0, "Max"=0.0, "Coerced"=0.0, "Command"="CFIL"}, {"Name"="RSZVL_VAL_MPOW_FTYPE_RRC", "Discrete or Min"=2.0, "Max"=0.0, "Coerced"=0.0, "Command"="RRC"}]}, {"Name"="rszvl_rngPct", "Type"=0, "Min?"=TRUE, "Max?"=TRUE, "Entries"=[{"Name"="", "Discrete or Min"=0.0, "Max"=100.0, "Coerced"=0.0, "Command"=""}]}, {"Name"="rszvl_rngRefLevelOffset", "Type"=0, "Min?"=TRUE, "Max?"=TRUE, "Entries"=[{"Name"="", "Discrete or Min"=-100.0, "Max"=100.0, "Coerced"=0.0, "Command"=""}]}, {"Name"="rszvl_rngRefLevel", "Type"=0, "Min?"=TRUE, "Max?"=TRUE, "Entries"=[{"Name"="", "Discrete or Min"=-200.0, "Max"=200.0, "Coerced"=0.0, "Command"=""}]}, {"Name"="rszvl_rngVBW", "Type"=0, "Min?"=TRUE, "Max?"=TRUE, "Entries"=[{"Name"="", "Discrete or Min"=1.0, "Max"=10000000.0, "Coerced"=0.0, "Command"=""}]}, {"Name"="rszvl_rngFreqOffset", "Type"=0, "Min?"=TRUE, "Max?"=TRUE, "Entries"=[{"Name"="", "Discrete or Min"=-100000000000.0, "Max"=100000000000.0, "Coerced"=0.0, "Command"=""}]}, {"Name"="rszvl_rngSweepCount", "Type"=0, "Min?"=TRUE, "Max?"=TRUE, "Entries"=[{"Name"="", "Discrete or Min"=0.0, "Max"=32767.0, "Coerced"=0.0, "Command"=""}]}, {"Name"="rszvl_rngDISPConfPowSave", "Type"=0, "Min?"=TRUE, "Max?"=TRUE, "Entries"=[{"Name"="", "Discrete or Min"=1.0, "Max"=60.0, "Coerced"=0.0, "Command"=""}]}, {"Name"="rszvl_rngTrace", "Type"=0, "Min?"=TRUE, "Max?"=TRUE, "Entries"=[{"Name"="", "Discrete or Min"=1.0, "Max"=6.0, "Coerced"=0.0, "Command"=""}]}, {"Name"="rszvl_rngExtGateDelay", "Type"=0, "Min?"=TRUE, "Max?"=TRUE, "Entries"=[{"Name"="", "Discrete or Min"=0.0, "Max"=100.0, "Coerced"=0.0, "Command"=""}]}, {"Name"="rszvl_rngLimits", "Type"=0, "Min?"=TRUE, "Max?"=TRUE, "Entries"=[{"Name"="", "Discrete or Min"=1.0, "Max"=8.0, "Coerced"=0.0, "Command"=""}]}, {"Name"="rszvl_rngLimitOffset", "Type"=0, "Min?"=TRUE, "Max?"=TRUE, "Entries"=[{"Name"="", "Discrete or Min"=-300000000000.0, "Max"=300000000000.0, "Coerced"=0.0, "Command"=""}]}, {"Name"="rszvl_rngLimitMargin", "Type"=0, "Min?"=TRUE, "Max?"=TRUE, "Entries"=[{"Name"="", "Discrete or Min"=0.0, "Max"=200.0, "Coerced"=0.0, "Command"=""}]}, {"Name"="rszvl_rngDISPAmplitudeRang", "Type"=0, "Min?"=TRUE, "Max?"=TRUE, "Entries"=[{"Name"="", "Discrete or Min"=10.0, "Max"=200.0, "Coerced"=0.0, "Command"=""}]}, {"Name"="rszvl_rngSwePoints", "Type"=0, "Min?"=TRUE, "Max?"=TRUE, "Entries"=[{"Name"="", "Discrete or Min"=125.0, "Max"=32001.0, "Coerced"=0.0, "Command"=""}]}, {"Name"="rszvl_rngBandRatio", "Type"=0, "Min?"=TRUE, "Max?"=TRUE, "Entries"=[{"Name"="", "Discrete or Min"=0.0001, "Max"=1.0, "Coerced"=0.0, "Command"=""}]}, {"Name"="rszvl_rngMarkerPeakListCount", "Type"=0, "Min?"=TRUE, "Max?"=TRUE, "Entries"=[{"Name"="", "Discrete or Min"=0.0, "Max"=50.0, "Coerced"=0.0, "Command"=""}]}, {"Name"="rszvl_rngMarkerNdBDown", "Type"=0, "Min?"=TRUE, "Max?"=TRUE, "Entries"=[{"Name"="", "Discrete or Min"=-100.0, "Max"=100.0, "Coerced"=0.0, "Command"=""}]}, {"Name"="rszvl_rngMarkerDemodHoldoff", "Type"=0, "Min?"=TRUE, "Max?"=TRUE, "Entries"=[{"Name"="", "Discrete or Min"=0.01, "Max"=1000.0, "Coerced"=0.0, "Command"=""}]}, {"Name"="rszvl_rngStatNumSamples", "Type"=0, "Min?"=TRUE, "Max?"=TRUE, "Entries"=[{"Name"="", "Discrete or Min"=100.0, "Max"=1000000000.0, "Coerced"=0.0, "Command"=""}]}, {"Name"="rszvl_rngMeasStatUpperLimit", "Type"=0, "Min?"=TRUE, "Max?"=TRUE, "Entries"=[{"Name"="", "Discrete or Min"=1e-08, "Max"=1.0, "Coerced"=0.0, "Command"=""}]}, {"Name"="rszvl_rngMeasStatLowerLimit", "Type"=0, "Min?"=TRUE, "Max?"=TRUE, "Entries"=[{"Name"="", "Discrete or Min"=1e-09, "Max"=0.1, "Coerced"=0.0, "Command"=""}]}, {"Name"="rszvl_rngMeasHDISTNharm", "Type"=0, "Min?"=TRUE, "Max?"=TRUE, "Entries"=[{"Name"="", "Discrete or Min"=1.0, "Max"=10.0, "Coerced"=0.0, "Command"=""}]}, {"Name"="rszvl_rngSweepTime", "Type"=0, "Min?"=TRUE, "Max?"=TRUE, "Entries"=[{"Name"="", "Discrete or Min"=1e-06, "Max"=16000.0, "Coerced"=0.0, "Command"=""}]}, {"Name"="rszvl_rngSignalTrackThreshold", "Type"=0, "Min?"=TRUE, "Max?"=TRUE, "Entries"=[{"Name"="", "Discrete or Min"=-330.0, "Max"=30.0, "Coerced"=0.0, "Command"=""}]}, {"Name"="rszvl_rngTraceMathPosition", "Type"=0, "Min?"=TRUE, "Max?"=TRUE, "Entries"=[{"Name"="", "Discrete or Min"=-100.0, "Max"=200.0, "Coerced"=0.0, "Command"=""}]}, {"Name"="rszvl_rngTimeLinePos", "Type"=0, "Min?"=TRUE, "Max?"=TRUE, "Entries"=[{"Name"="", "Discrete or Min"=0.0, "Max"=1000.0, "Coerced"=0.0, "Command"=""}]}, {"Name"="rszvl_rngRBW", "Type"=0, "Min?"=TRUE, "Max?"=TRUE, "Entries"=[{"Name"="", "Discrete or Min"=10.0, "Max"=50000000.0, "Coerced"=0.0, "Command"=""}]}, {"Name"="rszvl_rngVbwRatio", "Type"=0, "Min?"=TRUE, "Max?"=TRUE, "Entries"=[{"Name"="", "Discrete or Min"=0.01, "Max"=1000.0, "Coerced"=0.0, "Command"=""}]}, {"Name"="rszvl_rngAvgCount", "Type"=0, "Min?"=TRUE, "Max?"=TRUE, "Entries"=[{"Name"="", "Discrete or Min"=0.0, "Max"=32767.0, "Coerced"=0.0, "Command"=""}]}, {"Name"="rszvl_rngExtMixerPorts", "Type"=0, "Min?"=TRUE, "Max?"=TRUE, "Entries"=[{"Name"="", "Discrete or Min"=2.0, "Max"=3.0, "Coerced"=0.0, "Command"=""}]}, {"Name"="rszvl_rngExtMixerHarmonic", "Type"=0, "Min?"=TRUE, "Max?"=TRUE, "Entries"=[{"Name"="", "Discrete or Min"=2.0, "Max"=64.0, "Coerced"=0.0, "Command"=""}]}, {"Name"="rszvl_rngExtMixerTreshold", "Type"=0, "Min?"=TRUE, "Max?"=TRUE, "Entries"=[{"Name"="", "Discrete or Min"=0.1, "Max"=100.0, "Coerced"=0.0, "Command"=""}]}, {"Name"="rszvl_rngChannelSpacing", "Type"=0, "Min?"=TRUE, "Max?"=TRUE, "Entries"=[{"Name"="", "Discrete or Min"=100.0, "Max"=2000000000.0, "Coerced"=0.0, "Command"=""}]}, {"Name"="rszvl_rngCarrSignNum", "Type"=0, "Min?"=TRUE, "Max?"=TRUE, "Entries"=[{"Name"="", "Discrete or Min"=1.0, "Max"=12.0, "Coerced"=0.0, "Command"=""}]}, {"Name"="rszvl_rngAdjChNum", "Type"=0, "Min?"=TRUE, "Max?"=TRUE, "Entries"=[{"Name"="", "Discrete or Min"=0.0, "Max"=12.0, "Coerced"=0.0, "Command"=""}]}, {"Name"="rszvl_rngChannelBandwidth", "Type"=0, "Min?"=TRUE, "Max?"=TRUE, "Entries"=[{"Name"="", "Discrete or Min"=100.0, "Max"=1000000000.0, "Coerced"=0.0, "Command"=""}]}, {"Name"="rszvl_rngAdjRefTxChann", "Type"=0, "Min?"=TRUE, "Max?"=TRUE, "Entries"=[{"Name"="", "Discrete or Min"=1.0, "Max"=12.0, "Coerced"=0.0, "Command"=""}]}, {"Name"="rszvl_rngPowPct", "Type"=0, "Min?"=TRUE, "Max?"=TRUE, "Entries"=[{"Name"="", "Discrete or Min"=10.0, "Max"=99.9, "Coerced"=0.0, "Command"=""}]}, {"Name"="rszvl_rngExtGateLength", "Type"=0, "Min?"=TRUE, "Max?"=TRUE, "Entries"=[{"Name"="", "Discrete or Min"=1.25e-07, "Max"=100.0, "Coerced"=0.0, "Command"=""}]}, {"Name"="rszvl_rngTrigIFPowerLevel", "Type"=0, "Min?"=TRUE, "Max?"=TRUE, "Entries"=[{"Name"="", "Discrete or Min"=-50.0, "Max"=-10.0, "Coerced"=0.0, "Command"=""}]}, {"Name"="rszvl_rngTriggerDelay", "Type"=0, "Min?"=TRUE, "Max?"=TRUE, "Entries"=[{"Name"="", "Discrete or Min"=-100.0, "Max"=100.0, "Coerced"=0.0, "Command"=""}]}, {"Name"="rszvl_rngSpeakerVolume", "Type"=0, "Min?"=TRUE, "Max?"=TRUE, "Entries"=[{"Name"="", "Discrete or Min"=0.0, "Max"=1.0, "Coerced"=0.0, "Command"=""}]}, {"Name"="rszvl_rngLinkFactor", "Type"=0, "Min?"=TRUE, "Max?"=TRUE, "Entries"=[{"Name"="", "Discrete or Min"=1.0, "Max"=100.0, "Coerced"=0.0, "Command"=""}]}, {"Name"="rszvl_rngBias", "Type"=0, "Min?"=TRUE, "Max?"=TRUE, "Entries"=[{"Name"="", "Discrete or Min"=-0.01, "Max"=0.01, "Coerced"=0.0, "Command"=""}]}, {"Name"="rszvl_rngSEListRangeLimit", "Type"=0, "Min?"=TRUE, "Max?"=TRUE, "Entries"=[{"Name"="", "Discrete or Min"=-200.0, "Max"=200.0, "Coerced"=0.0, "Command"=""}]}, {"Name"="rszvl_rngIFPowOffset", "Type"=0, "Min?"=TRUE, "Max?"=TRUE, "Entries"=[{"Name"="", "Discrete or Min"=1.5e-07, "Max"=1000.0, "Coerced"=0.0, "Command"=""}]}, {"Name"="rszvl_rngIFPowHyst", "Type"=0, "Min?"=TRUE, "Max?"=TRUE, "Entries"=[{"Name"="", "Discrete or Min"=3.0, "Max"=50.0, "Coerced"=0.0, "Command"=""}]}, {"Name"="rszvl_rngTriggerTimeInterval", "Type"=0, "Min?"=TRUE, "Max?"=TRUE, "Entries"=[{"Name"="", "Discrete or Min"=0.1, "Max"=5000.0, "Coerced"=0.0, "Command"=""}]}, {"Name"="rszvl_rngAttenuationRangeTable", "Type"=1, "Min?"=FALSE, "Max?"=FALSE, "Entries"=[{"Name"="", "Discrete or Min"=0.0, "Max"=0.0, "Coerced"=0.0, "Command"=""}, {"Name"="", "Discrete or Min"=0.0, "Max"=0.0, "Coerced"=5.0, "Command"=""}, {"Name"="", "Discrete or Min"=0.0, "Max"=0.0, "Coerced"=10.0, "Command"=""}, {"Name"="", "Discrete or Min"=0.0, "Max"=0.0, "Coerced"=15.0, "Command"=""}, {"Name"="", "Discrete or Min"=0.0, "Max"=0.0, "Coerced"=20.0, "Command"=""}, {"Name"="", "Discrete or Min"=0.0, "Max"=0.0, "Coerced"=25.0, "Command"=""}, {"Name"="", "Discrete or Min"=0.0, "Max"=0.0, "Coerced"=30.0, "Command"=""}, {"Name"="", "Discrete or Min"=0.0, "Max"=0.0, "Coerced"=35.0, "Command"=""}, {"Name"="", "Discrete or Min"=0.0, "Max"=0.0, "Coerced"=40.0, "Command"=""}, {"Name"="", "Discrete or Min"=0.0, "Max"=0.0, "Coerced"=45.0, "Command"=""}, {"Name"="", "Discrete or Min"=0.0, "Max"=0.0, "Coerced"=50.0, "Command"=""}, {"Name"="", "Discrete or Min"=0.0, "Max"=0.0, "Coerced"=55.0, "Command"=""}, {"Name"="", "Discrete or Min"=0.0, "Max"=0.0, "Coerced"=60.0, "Command"=""}, {"Name"="", "Discrete or Min"=0.0, "Max"=0.0, "Coerced"=65.0, "Command"=""}, {"Name"="", "Discrete or Min"=0.0, "Max"=0.0, "Coerced"=70.0, "Command"=""}, {"Name"="", "Discrete or Min"=0.0, "Max"=0.0, "Coerced"=75.0, "Command"=""}]}, {"Name"="rszvl_rngInputImpedance", "Type"=1, "Min?"=FALSE, "Max?"=FALSE, "Entries"=[{"Name"="", "Discrete or Min"=0.0, "Max"=0.0, "Coerced"=50.0, "Command"=""}, {"Name"="", "Discrete or Min"=0.0, "Max"=0.0, "Coerced"=75.0, "Command"=""}]}, {"Name"="rszvl_rngInpAmptEattMan", "Type"=1, "Min?"=FALSE, "Max?"=FALSE, "Entries"=[{"Name"="", "Discrete or Min"=0.0, "Max"=0.0, "Coerced"=0.0, "Command"=""}, {"Name"="", "Discrete or Min"=0.0, "Max"=0.0, "Coerced"=5.0, "Command"=""}, {"Name"="", "Discrete or Min"=0.0, "Max"=0.0, "Coerced"=10.0, "Command"=""}, {"Name"="", "Discrete or Min"=0.0, "Max"=0.0, "Coerced"=15.0, "Command"=""}, {"Name"="", "Discrete or Min"=0.0, "Max"=0.0, "Coerced"=20.0, "Command"=""}, {"Name"="", "Discrete or Min"=0.0, "Max"=0.0, "Coerced"=25.0, "Command"=""}, {"Name"="", "Discrete or Min"=0.0, "Max"=0.0, "Coerced"=30.0, "Command"=""}]}, {"Name"="rszvl_rngFreqCountRes", "Type"=1, "Min?"=FALSE, "Max?"=FALSE, "Entries"=[{"Name"="", "Discrete or Min"=0.0, "Max"=0.0, "Coerced"=0.1, "Command"=""}, {"Name"="", "Discrete or Min"=0.0, "Max"=0.0, "Coerced"=1.0, "Command"=""}, {"Name"="", "Discrete or Min"=0.0, "Max"=0.0, "Coerced"=10.0, "Command"=""}, {"Name"="", "Discrete or Min"=0.0, "Max"=0.0, "Coerced"=100.0, "Command"=""}, {"Name"="", "Discrete or Min"=0.0, "Max"=0.0, "Coerced"=1000.0, "Command"=""}, {"Name"="", "Discrete or Min"=0.0, "Max"=0.0, "Coerced"=10000.0, "Command"=""}]}, {"Name"="rszvl_rngExtMixerLoPower", "Type"=1, "Min?"=FALSE, "Max?"=FALSE, "Entries"=[{"Name"="", "Discrete or Min"=0.0, "Max"=0.0, "Coerced"=13.0, "Command"=""}, {"Name"="", "Discrete or Min"=0.0, "Max"=0.0, "Coerced"=13.1, "Command"=""}, {"Name"="", "Discrete or Min"=0.0, "Max"=0.0, "Coerced"=13.2, "Command"=""}, {"Name"="", "Discrete or Min"=0.0, "Max"=0.0, "Coerced"=13.3, "Command"=""}, {"Name"="", "Discrete or Min"=0.0, "Max"=0.0, "Coerced"=13.4, "Command"=""}, {"Name"="", "Discrete or Min"=0.0, "Max"=0.0, "Coerced"=13.5, "Command"=""}, {"Name"="", "Discrete or Min"=0.0, "Max"=0.0, "Coerced"=13.6, "Command"=""}, {"Name"="", "Discrete or Min"=0.0, "Max"=0.0, "Coerced"=13.7, "Command"=""}, {"Name"="", "Discrete or Min"=0.0, "Max"=0.0, "Coerced"=13.8, "Command"=""}, {"Name"="", "Discrete or Min"=0.0, "Max"=0.0, "Coerced"=13.9, "Command"=""}, {"Name"="", "Discrete or Min"=0.0, "Max"=0.0, "Coerced"=14.0, "Command"=""}, {"Name"="", "Discrete or Min"=0.0, "Max"=0.0, "Coerced"=14.1, "Command"=""}, {"Name"="", "Discrete or Min"=0.0, "Max"=0.0, "Coerced"=14.2, "Command"=""}, {"Name"="", "Discrete or Min"=0.0, "Max"=0.0, "Coerced"=14.3, "Command"=""}, {"Name"="", "Discrete or Min"=0.0, "Max"=0.0, "Coerced"=14.4, "Command"=""}, {"Name"="", "Discrete or Min"=0.0, "Max"=0.0, "Coerced"=14.5, "Command"=""}, {"Name"="", "Discrete or Min"=0.0, "Max"=0.0, "Coerced"=14.6, "Command"=""}, {"Name"="", "Discrete or Min"=0.0, "Max"=0.0, "Coerced"=14.7, "Command"=""}, {"Name"="", "Discrete or Min"=0.0, "Max"=0.0, "Coerced"=14.8, "Command"=""}, {"Name"="", "Discrete or Min"=0.0, "Max"=0.0, "Coerced"=14.9, "Command"=""}, {"Name"="", "Discrete or Min"=0.0, "Max"=0.0, "Coerced"=15.0, "Command"=""}, {"Name"="", "Discrete or Min"=0.0, "Max"=0.0, "Coerced"=15.1, "Command"=""}, {"Name"="", "Discrete or Min"=0.0, "Max"=0.0, "Coerced"=15.2, "Command"=""}, {"Name"="", "Discrete or Min"=0.0, "Max"=0.0, "Coerced"=15.3, "Command"=""}, {"Name"="", "Discrete or Min"=0.0, "Max"=0.0, "Coerced"=15.4, "Command"=""}, {"Name"="", "Discrete or Min"=0.0, "Max"=0.0, "Coerced"=15.5, "Command"=""}, {"Name"="", "Discrete or Min"=0.0, "Max"=0.0, "Coerced"=15.6, "Command"=""}, {"Name"="", "Discrete or Min"=0.0, "Max"=0.0, "Coerced"=15.7, "Command"=""}, {"Name"="", "Discrete or Min"=0.0, "Max"=0.0, "Coerced"=15.8, "Command"=""}, {"Name"="", "Discrete or Min"=0.0, "Max"=0.0, "Coerced"=15.9, "Command"=""}, {"Name"="", "Discrete or Min"=0.0, "Max"=0.0, "Coerced"=16.0, "Command"=""}, {"Name"="", "Discrete or Min"=0.0, "Max"=0.0, "Coerced"=16.1, "Command"=""}, {"Name"="", "Discrete or Min"=0.0, "Max"=0.0, "Coerced"=16.2, "Command"=""}, {"Name"="", "Discrete or Min"=0.0, "Max"=0.0, "Coerced"=16.3, "Command"=""}, {"Name"="", "Discrete or Min"=0.0, "Max"=0.0, "Coerced"=16.4, "Command"=""}, {"Name"="", "Discrete or Min"=0.0, "Max"=0.0, "Coerced"=16.5, "Command"=""}, {"Name"="", "Discrete or Min"=0.0, "Max"=0.0, "Coerced"=16.6, "Command"=""}, {"Name"="", "Discrete or Min"=0.0, "Max"=0.0, "Coerced"=16.7, "Command"=""}, {"Name"="", "Discrete or Min"=0.0, "Max"=0.0, "Coerced"=16.8, "Command"=""}, {"Name"="", "Discrete or Min"=0.0, "Max"=0.0, "Coerced"=16.9, "Command"=""}, {"Name"="", "Discrete or Min"=0.0, "Max"=0.0, "Coerced"=17.0, "Command"=""}]}, {"Name"="rszvl_rngPmetAverCount", "Type"=1, "Min?"=FALSE, "Max?"=FALSE, "Entries"=[{"Name"="", "Discrete or Min"=0.0, "Max"=0.0, "Coerced"=1.0, "Command"=""}, {"Name"="", "Discrete or Min"=0.0, "Max"=0.0, "Coerced"=2.0, "Command"=""}, {"Name"="", "Discrete or Min"=0.0, "Max"=0.0, "Coerced"=4.0, "Command"=""}, {"Name"="", "Discrete or Min"=0.0, "Max"=0.0, "Coerced"=8.0, "Command"=""}, {"Name"="", "Discrete or Min"=0.0, "Max"=0.0, "Coerced"=16.0, "Command"=""}, {"Name"="", "Discrete or Min"=0.0, "Max"=0.0, "Coerced"=32.0, "Command"=""}, {"Name"="", "Discrete or Min"=0.0, "Max"=0.0, "Coerced"=64.0, "Command"=""}, {"Name"="", "Discrete or Min"=0.0, "Max"=0.0, "Coerced"=128.0, "Command"=""}, {"Name"="", "Discrete or Min"=0.0, "Max"=0.0, "Coerced"=256.0, "Command"=""}]}, {"Name"="rszvl_rngServiceCombFrequency", "Type"=2, "Min?"=FALSE, "Max?"=FALSE, "Entries"=[{"Name"="RSZVL_VAL_SERV_COMB_FREQ_COMB1", "Discrete or Min"=0.0, "Max"=0.0, "Coerced"=0.0, "Command"="COMB1"}, {"Name"="RSZVL_VAL_SERV_COMB_FREQ_COMB64", "Discrete or Min"=1.0, "Max"=0.0, "Coerced"=0.0, "Command"="COMB64"}, {"Name"="RSZVL_VAL_SERV_COMB_FREQ_COMB65", "Discrete or Min"=2.0, "Max"=0.0, "Coerced"=0.0, "Command"="COMB65"}]}, {"Name"="rszvl_rngTraceSpacing", "Type"=2, "Min?"=FALSE, "Max?"=FALSE, "Entries"=[{"Name"="RSZVL_VAL_TRACE_SPACE_LIN", "Discrete or Min"=0.0, "Max"=0.0, "Coerced"=0.0, "Command"="LIN"}, {"Name"="RSZVL_VAL_TRACE_SPACE_LOG", "Discrete or Min"=1.0, "Max"=0.0, "Coerced"=0.0, "Command"="LOG"}, {"Name"="RSZVL_VAL_TRACE_SPACE_PCT", "Discrete or Min"=2.0, "Max"=0.0, "Coerced"=0.0, "Command"="PERC"}, {"Name"="RSZVL_VAL_TRACE_SPACE_LDB", "Discrete or Min"=3.0, "Max"=0.0, "Coerced"=0.0, "Command"="LDB"}]}, {"Name"="rszvl_rngNWANumberOfSweeps", "Type"=0, "Min?"=TRUE, "Max?"=TRUE, "Entries"=[{"Name"="", "Discrete or Min"=1.0, "Max"=999.0, "Coerced"=0.0, "Command"=""}]}, {"Name"="rszvl_rngNWAAvgCount", "Type"=0, "Min?"=TRUE, "Max?"=TRUE, "Entries"=[{"Name"="", "Discrete or Min"=1.0, "Max"=1000.0, "Coerced"=0.0, "Command"=""}]}, {"Name"="rszvl_rngNWARBW", "Type"=0, "Min?"=TRUE, "Max?"=TRUE, "Entries"=[{"Name"="", "Discrete or Min"=10.0, "Max"=500000.0, "Coerced"=0.0, "Command"=""}]}, {"Name"="rszvl_rngNWASwePoints", "Type"=0, "Min?"=TRUE, "Max?"=TRUE, "Entries"=[{"Name"="", "Discrete or Min"=2.0, "Max"=4001.0, "Coerced"=0.0, "Command"=""}]}, {"Name"="rszvl_rngNWASourcePort", "Type"=0, "Min?"=TRUE, "Max?"=TRUE, "Entries"=[{"Name"="", "Discrete or Min"=1.0, "Max"=2.0, "Coerced"=0.0, "Command"=""}]}, {"Name"="rszvl_rngNWASweepType", "Type"=2, "Min?"=FALSE, "Max?"=FALSE, "Entries"=[{"Name"="RSZVL_VAL_SWE_TYPE_LIN", "Discrete or Min"=0.0, "Max"=0.0, "Coerced"=0.0, "Command"="LIN"}, {"Name"="RSZVL_VAL_SWE_TYPE_LOG", "Discrete or Min"=1.0, "Max"=0.0, "Coerced"=0.0, "Command"="LOG"}, {"Name"="RSZVL_VAL_SWE_TYPE_SEG", "Discrete or Min"=2.0, "Max"=0.0, "Coerced"=0.0, "Command"="SEGM"}]}, {"Name"="rszvl_rngNWASweepMeasDelay", "Type"=0, "Min?"=TRUE, "Max?"=TRUE, "Entries"=[{"Name"="", "Discrete or Min"=0.0, "Max"=317.9551, "Coerced"=0.0, "Command"=""}]}, {"Name"="rszvl_rngNWASegmentSelectSweepTime", "Type"=2, "Min?"=FALSE, "Max?"=FALSE, "Entries"=[{"Name"="RSZVL_VAL_SEG_SWE_TIME_SWT", "Discrete or Min"=0.0, "Max"=0.0, "Coerced"=0.0, "Command"="SWT"}, {"Name"="RSZVL_VAL_SEG_SWE_TIME_DWEL", "Discrete or Min"=1.0, "Max"=0.0, "Coerced"=0.0, 
